vi "1st.vi"() -> ()   [LabVIEW 2014]
uses:
  Event_class/EventMsg.lvclass
panel:
  out "data":string
  out "Msg":string
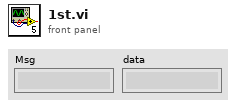
[diagram p1: front panel]
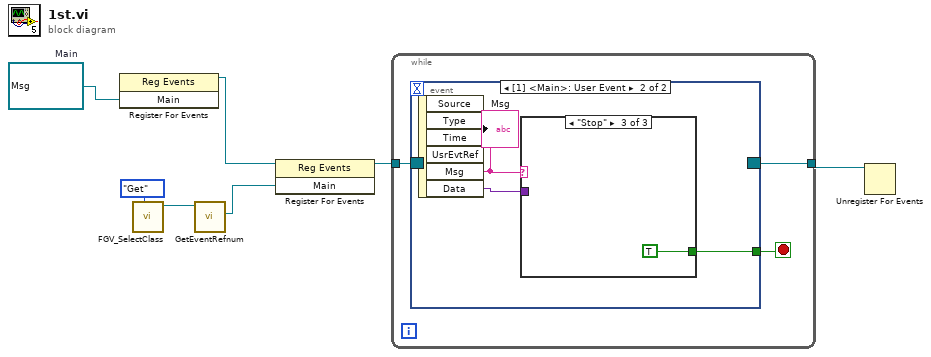
[diagram p0: block diagram]
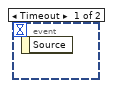
[diagram p2: hidden frame]
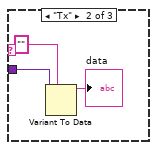
[diagram p4: hidden frame]
diagram:
  w4 = refnum<user-event> refnum  # Main
  n1 = register-events(w4) -> (reference out=w3:refnum<event-registration>)  [unwired: 2 in, 1 out]
  n2 = call "FGV_SelectClass.vi"("Action"=enum16{"Set", "Get"}."Get") -> ("EventMsg.lvclass 2"=w6:refnum<class "EventMsg.lvclass">)  [unwired: 10 in]
  n3 = call-dynamic "GetEventRefnum.vi"("object in"=w6) -> ("MsgEvent"=w5:refnum<user-event>)  [unwired: 8 in, 2 out]
  n4 = register-events(reference=w3, w5) -> (reference out=w2:refnum<event-registration>)  [unwired: 1 in, 1 out]
  n5 = while {
    tunnel: w2 -> [w10]
    tunnel: [w9] -> w1
    stop <- w8 stop-if-true
    n6 = event shown="[1] <Main>: User Event" {
      selector: w10 -> [_ _]
      dyn-events: [_ _] -> w9
      timeout: _ -> [_ _]
      tunnel: [_ w12] -> w8
      event Timeout {
        n7 = event-data() -> ()  [unwired: 1 in, 1 out]
      }
      event User Event {
        n8 = event-data() -> ("Msg"=w13:string, "Data"=w11:variant)  [unwired: 1 in, 4 out]
        "Msg" <- w13
        n9 = case shown="\"Stop\"" w13 {
          tunnel: [_ _ TRUE] -> w12
          tunnel: w11 -> [_ w16 _]
          frame "False", Default {
          }
          frame "Tx" {
            n10 = Variant To Data(type="", Variant=w16) -> (data=→"data":string)  [unwired: 1 in, 1 out]
          }
          frame "Stop" {
          }
        }
      }
    }
  }
  n11 = Unregister For Events(event registration refnum=w1) -> ()  [unwired: 1 in, 1 out]
